vi "Vision Processing.vi"(4 "error in (no error)":errorcluster) -> ()   [LabVIEW 2011]
doc: "This VI runs in parallel to other tasks. It gets images from the camera, processes them for color or shape and use that information to affect robot behavior."
uses:
  <vilib>/Rock Robotics/WPI/Camera/WPI_CameraImageSize.ctl
  <vilib>/Rock Robotics/WPI/Camera/WPI_CameraFrameRate.ctl
  <vilib>/Rock Robotics/WPI/Camera/WPI_CameraExposure Priority Values.ctl
  <vilib>/Rock Robotics/WPI/Camera/WPI_CameraExposure Values.ctl
  <vilib>/Rock Robotics/WPI/Camera/WPI_CameraWhite Balance Values.ctl
  Robot Global Data.vi
  <vilib>/Rock Robotics/WPI/RobotDrive/WPI_RobotDriveArcadeDrive_Standard(NoSaturation).vi
  <vilib>/vision/NI_Vision_Development_Module.lvlib
panel:
  out "max index(es)":i32[](array[numeric])
  out "Loop Speed":u32(knob) scale=100.0..1000.0
  out "Distance":dbl(graph)
  out "Y Error":dbl(graph)
  out "Distance":dbl
  in  "Servo Tilt Gain":dbl=100.0
  out "error out":errorcluster
  out "ServoPosition":dbl
  out "Image Size":T1
  out "X Error":dbl(graph)
  out "X Error":dbl
  in  "Turning Gain":dbl=0.01
  in  "Tracking?":bool
  out "Particle Measurements (Pixels)":dbl[][](array[numeric]) format="%.2f"
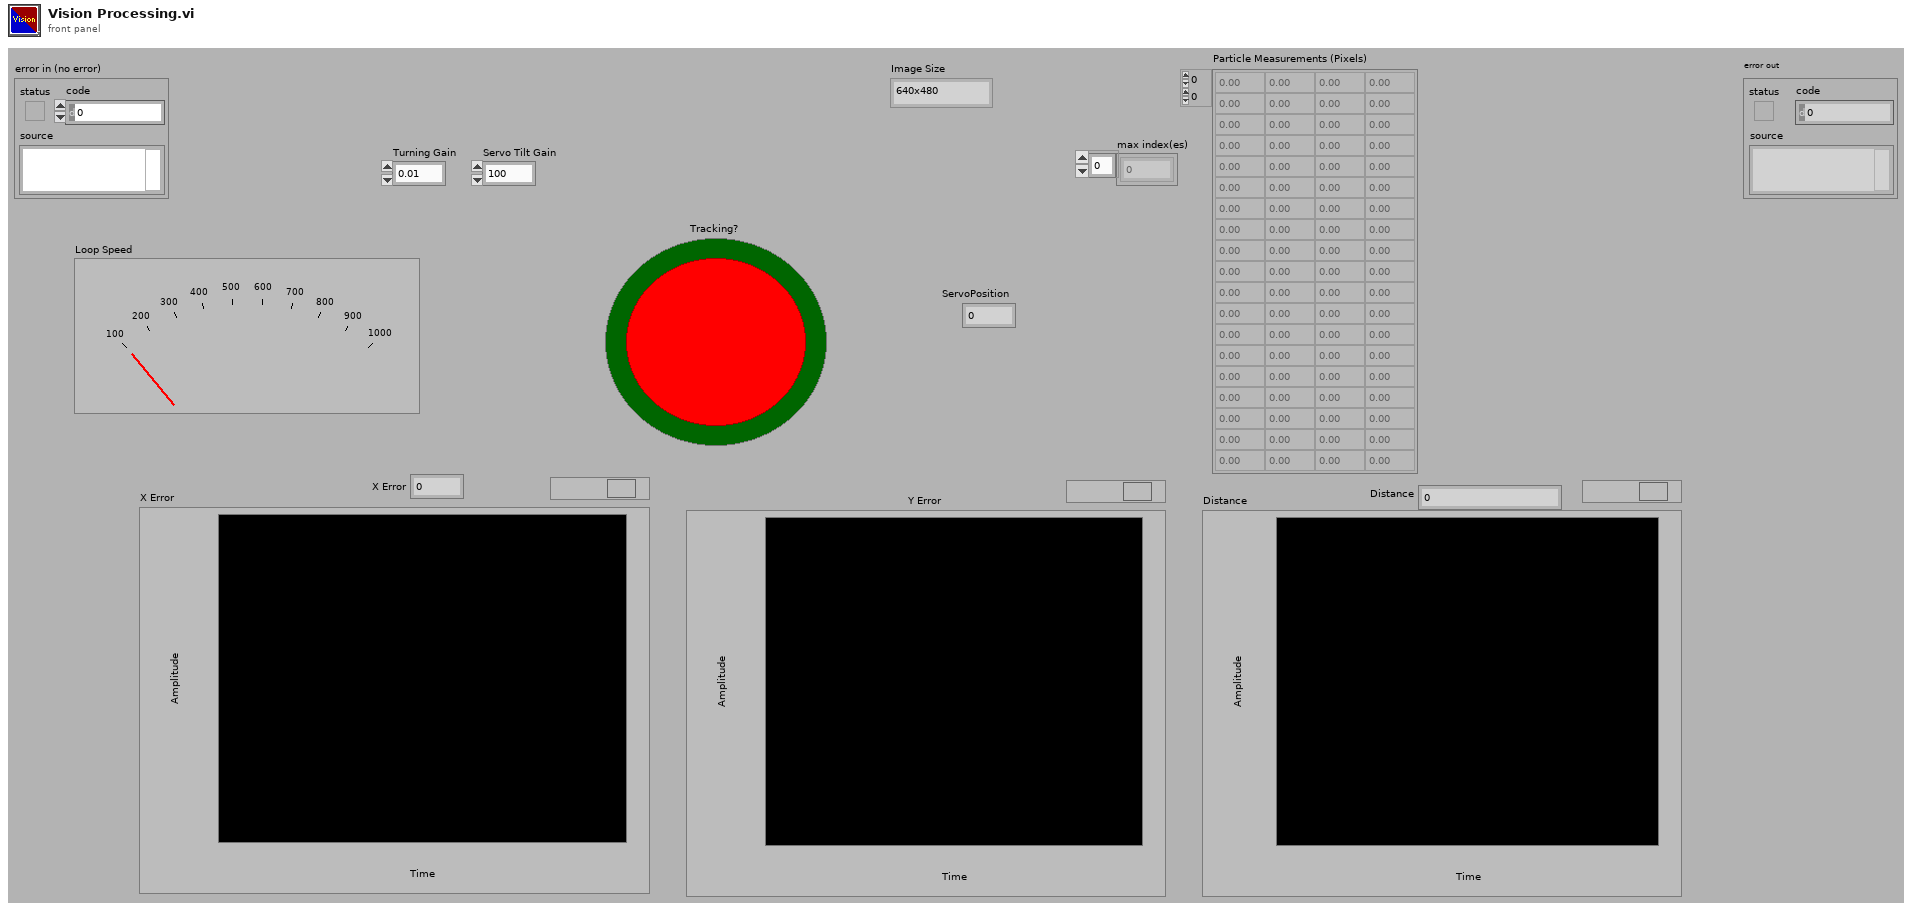
[diagram p1: front panel]
types:
  T1 = typedef "WPI_CameraImageSize.ctl" = enum16{"640x480", "320x240", "160x120"}
  T2 = typedef "Image Type" = u32
  T3 = typedef "WPI_CameraDevRef.ctl" = cluster{"Camera Address":string, "CameraStatus":errorcluster, "Acquire Image Notifier":refnum<notifier>}
  T4 = typedef "WPI_ServoDeviceRef.ctl" = cluster{"DeviceStatus":errorcluster, "Digital Module":T5, "PWM Channel":T6, "DeadBand":T7}
  T5 = typedef "FPGA_TypedefDigitalModule.ctl" = enum16{"Digital Module 1", "Digital Module 2"}
  T6 = typedef "FPGA_DIOPWMChannel.ctl" = enum8{"PWM 1", "PWM 2", "PWM 3", "PWM 4", "PWM 5", "PWM 6", "PWM 7", "PWM 8", "PWM 9", "PWM 10", "Invalid"}
  T7 = typedef "WPI_PWMDeadband.ctl" = cluster{"Name":string, "maxPositivePwm":i32, "minPositivePwm":i32, "centerPwm":i32, "maxNegativePwm":i32, "minNegativePwm":i32, "angularRange":u16}
  T8 = typedef "IMAQ Image.ctl" = refnum<image>
  T9 = enum32{"AutoM", "Close", "Dilate", "Erode", "Gradient", "Gradient out", "Gradient in", "Hit miss", "Open", "PClose", "POpen", "Thick", "Thin"}
  T10 = typedef "WPI_CameraFrameRate.ctl" = u32
  T11 = typedef "WPI_CameraExposure Priority Values.ctl" = enum16{"None", "Prioritize frame rate", "Prioritize image quality"}
  T12 = typedef "WPI_CameraExposure Values.ctl" = enum16{"Auto", "Flicker-free 50 Hz", "Flicker-free 60 Hz", "Hold current"}
  T13 = typedef "WPI_CameraWhite Balance Values.ctl" = enum16{"Auto", "Fixed indoor", "Fixed outdoor 1", "Fixed outdoor 2", "Fixed fluorescent 1", "Fixed fluorescent 2", "Hold current"}
  T14 = typedef "WPI_RobotDriveDevRef.ctl" = cluster{"DevStatus":errorcluster, "Motors[]":T15[], "Square Inputs":bool, "Max Output":dbl, "Isochronous":bool}
  T15 = typedef "WPI_MotorControlDeviceRef.ctl" = cluster{"DeviceStatus":errorcluster, "Type":enum16{"PWM", "CAN"}, "PWM":cluster{"Digital Module":T5, "PWM Channel":T6, "DeadBand":T7}, "CAN":cluster{"Device Number":u8, "Control Mode":T16, "Semaphore":T17, "Max Vout":dbl}, "Invert":bool, "TransformRef":T18, "InvTransformRef":T18}
  T16 = typedef "WPI_CANJaguar_ControlMode.ctl" = enum8{"Percent VBus", "Current", "Speed", "Position", "Voltage"}
  T17 = typedef "Semaphore RefNum" = refnum<k1>
  T18 = typedef "WPI_PWMTransform_ConPane.ctl" = refnum<vi>
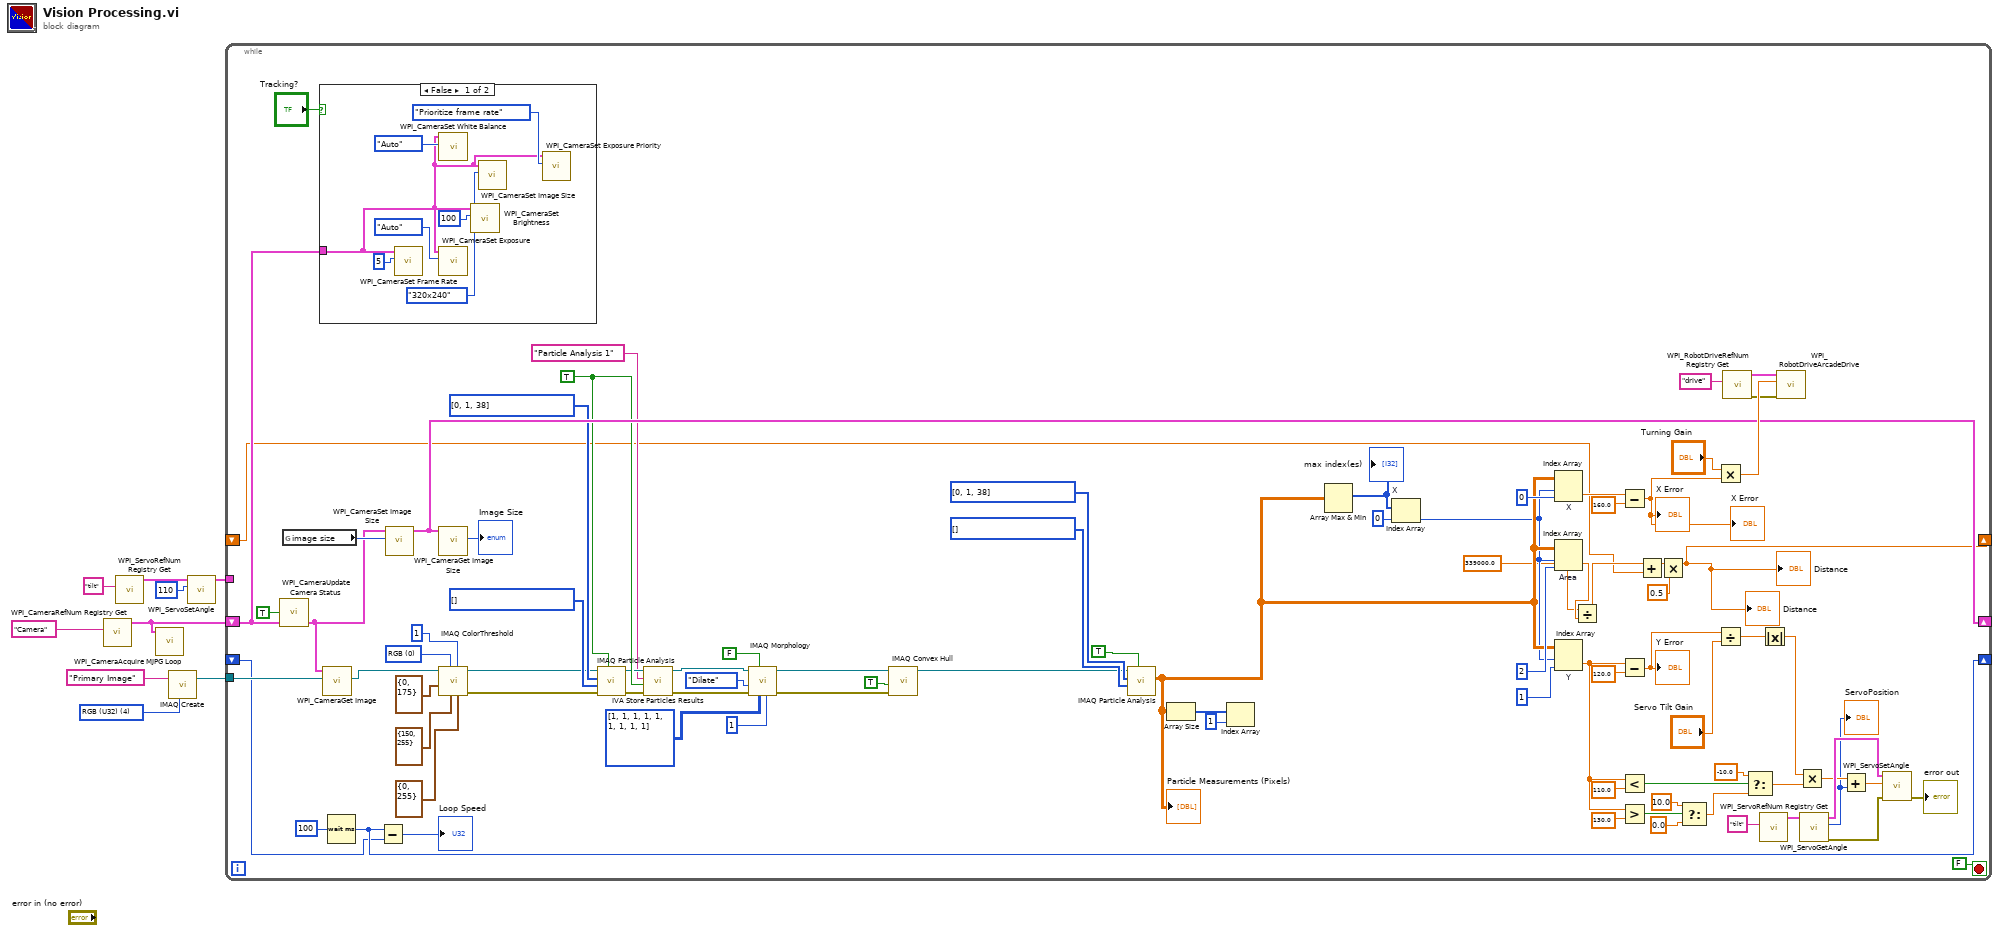
[diagram p0: block diagram]
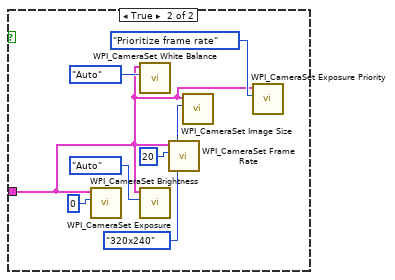
[diagram p2: hidden frame]
diagram:
  w9 = T2 4 items=["Grayscale (U8)", "Grayscale (I16)", "Grayscale (SGL)", "Complex (CSG)", "RGB (U32)", "HSL (U32)", "RGB (U64)"] ("Image Type")
  n1 = call <vilib>:"WPI_CameraRefNum Registry Get.vi"("refnum name"="Camera") -> ("CameraDevRef"=w5:T3)  [unwired: 1 in, 9 out]
  n2 = call <vilib>:"WPI_ServoRefNum Registry Get.vi"("refnum name"="tilt") -> ("ServoDeviceRef"=w2:T4)  [unwired: 9 in, 1 out]
  n3 = call <vilib>:"WPI_CameraAcquire MJPG Loop.vi"("CameraDevRef"=w5) -> ()  [unwired: 11 in]
  n4 = call "IMAQ Create"("Image Name"="Primary Image", "Image Type"=w9) -> ("New Image"=w7:T8)  [unwired: 2 in, 2 out]
  n5 = call <vilib>:"WPI_ServoSetAngle.vi"("Angle"=110, "ServoDeviceRef"=w2) -> ("ServoDeviceRef"=w1:T4)  [unwired: 8 in, 1 out]
  n6 = while {
    shift-right: [w74] -> _
    shift-left: w5 -> [w93]
    tunnel: w7 -> [w73]
    tunnel: w1 -> [_]
    shift-right: [w50] -> _
    shift-left: _ -> [w49]
    shift-right: [w12] -> _
    shift-left: _ -> [w10]
    stop <- FALSE stop-if-true
    w24 = i32[] [] items=["Center of Mass X", "Center of Mass Y", "First Pixel X", "First Pixel Y", "Bounding Rect Left", "Bounding Rect Top", "Bounding Rect Right", "Bounding Rect Bottom", "Max Feret Diameter Start X", "Max Feret Diameter Start Y", "Max Feret Diameter End X", "Max Feret Diameter End Y", "Max Horiz. Segment Length Left", "Max Horiz. Segment Length Right", "Max Horiz. Segment Length Row", "-", "Bounding Rect Width", "Bounding Rect Height", "Bounding Rect Diagonal", "Perimeter", "Convex Hull Perimeter", "Holes' Perimeter", "Max Feret Diameter", "Equivalent Ellipse Major Axis", "Equivalent Ellipse Minor Axis", "Equivalent Ellipse Minor Axis (Feret)", "Equivalent Rect Long Side", "Equivalent Rect Short Side", "Equivalent Rect Diagonal", "Equivalent Rect Short Side (Feret)", "Average Horiz. Segment Length", "Average Vert. Segment Length", "Hydraulic Radius", "Waddel Disk Diameter", "-", "Area", "Holes' Area", "Particle & Holes' Area", "Convex Hull Area", "Image Area", "-", "Number of Holes", "Number of Horiz. Segments", "Number of Vert. Segments", "-", "Orientation", "Max Feret Diameter Orientation", "-", "% Area/Image Area", "% Area/(Particle & Holes' Area)", "Ratio of Equivalent Ellipse Axes", "Ratio of Equivalent Rect Sides", "-", "Elongation Factor", "Compactness Factor", "Heywood Circularity Factor", "Type Factor", "-", "Sum X", "Sum Y", "Sum XX", "Sum XY", "Sum YY", "Sum XXX", "Sum XXY", "Sum XYY", "Sum YYY", "-", "Moment of Inertia XX", "Moment of Inertia XY", "Moment of Inertia YY", "Moment of Inertia XXX", "Moment of Inertia XXY", "Moment of Inertia XYY", "Moment of Inertia YYY", "Norm. Moment of Inertia XX", "Norm. Moment of Inertia XY", "Norm. Moment of Inertia YY", "Norm. Moment of Inertia XXX", "Norm. Moment of Inertia XXY", "Norm. Moment of Inertia XYY", "Norm. Moment of Inertia YYY", "Hu Moment 1", "Hu Moment 2", "Hu Moment 3", "Hu Moment 4", "Hu Moment 5", "Hu Moment 6", "Hu Moment 7"] ("Real-World Measurements")
    w25 = i32[] [0, 1, 38] items=["Center of Mass X", "Center of Mass Y", "First Pixel X", "First Pixel Y", "Bounding Rect Left", "Bounding Rect Top", "Bounding Rect Right", "Bounding Rect Bottom", "Max Feret Diameter Start X", "Max Feret Diameter Start Y", "Max Feret Diameter End X", "Max Feret Diameter End Y", "Max Horiz. Segment Length Left", "Max Horiz. Segment Length Right", "Max Horiz. Segment Length Row", "-", "Bounding Rect Width", "Bounding Rect Height", "Bounding Rect Diagonal", "Perimeter", "Convex Hull Perimeter", "Holes' Perimeter", "Max Feret Diameter", "Equivalent Ellipse Major Axis", "Equivalent Ellipse Minor Axis", "Equivalent Ellipse Minor Axis (Feret)", "Equivalent Rect Long Side", "Equivalent Rect Short Side", "Equivalent Rect Diagonal", "Equivalent Rect Short Side (Feret)", "Average Horiz. Segment Length", "Average Vert. Segment Length", "Hydraulic Radius", "Waddel Disk Diameter", "-", "Area", "Holes' Area", "Particle & Holes' Area", "Convex Hull Area", "Image Area", "-", "Number of Holes", "Number of Horiz. Segments", "Number of Vert. Segments", "-", "Orientation", "Max Feret Diameter Orientation", "-", "% Area/Image Area", "% Area/(Particle & Holes' Area)", "Ratio of Equivalent Ellipse Axes", "Ratio of Equivalent Rect Sides", "-", "Elongation Factor", "Compactness Factor", "Heywood Circularity Factor", "Type Factor", "-", "Sum X", "Sum Y", "Sum XX", "Sum XY", "Sum YY", "Sum XXX", "Sum XXY", "Sum XYY", "Sum YYY", "-", "Moment of Inertia XX", "Moment of Inertia XY", "Moment of Inertia YY", "Moment of Inertia XXX", "Moment of Inertia XXY", "Moment of Inertia XYY", "Moment of Inertia YYY", "Norm. Moment of Inertia XX", "Norm. Moment of Inertia XY", "Norm. Moment of Inertia YY", "Norm. Moment of Inertia XXX", "Norm. Moment of Inertia XXY", "Norm. Moment of Inertia XYY", "Norm. Moment of Inertia YYY", "Hu Moment 1", "Hu Moment 2", "Hu Moment 3", "Hu Moment 4", "Hu Moment 5", "Hu Moment 6", "Hu Moment 7"] ("Pixel Measurements")
    w40 = i32[] [] items=["Center of Mass X", "Center of Mass Y", "First Pixel X", "First Pixel Y", "Bounding Rect Left", "Bounding Rect Top", "Bounding Rect Right", "Bounding Rect Bottom", "Max Feret Diameter Start X", "Max Feret Diameter Start Y", "Max Feret Diameter End X", "Max Feret Diameter End Y", "Max Horiz. Segment Length Left", "Max Horiz. Segment Length Right", "Max Horiz. Segment Length Row", "-", "Bounding Rect Width", "Bounding Rect Height", "Bounding Rect Diagonal", "Perimeter", "Convex Hull Perimeter", "Holes' Perimeter", "Max Feret Diameter", "Equivalent Ellipse Major Axis", "Equivalent Ellipse Minor Axis", "Equivalent Ellipse Minor Axis (Feret)", "Equivalent Rect Long Side", "Equivalent Rect Short Side", "Equivalent Rect Diagonal", "Equivalent Rect Short Side (Feret)", "Average Horiz. Segment Length", "Average Vert. Segment Length", "Hydraulic Radius", "Waddel Disk Diameter", "-", "Area", "Holes' Area", "Particle & Holes' Area", "Convex Hull Area", "Image Area", "-", "Number of Holes", "Number of Horiz. Segments", "Number of Vert. Segments", "-", "Orientation", "Max Feret Diameter Orientation", "-", "% Area/Image Area", "% Area/(Particle & Holes' Area)", "Ratio of Equivalent Ellipse Axes", "Ratio of Equivalent Rect Sides", "-", "Elongation Factor", "Compactness Factor", "Heywood Circularity Factor", "Type Factor", "-", "Sum X", "Sum Y", "Sum XX", "Sum XY", "Sum YY", "Sum XXX", "Sum XXY", "Sum XYY", "Sum YYY", "-", "Moment of Inertia XX", "Moment of Inertia XY", "Moment of Inertia YY", "Moment of Inertia XXX", "Moment of Inertia XXY", "Moment of Inertia XYY", "Moment of Inertia YYY", "Norm. Moment of Inertia XX", "Norm. Moment of Inertia XY", "Norm. Moment of Inertia YY", "Norm. Moment of Inertia XXX", "Norm. Moment of Inertia XXY", "Norm. Moment of Inertia XYY", "Norm. Moment of Inertia YYY", "Hu Moment 1", "Hu Moment 2", "Hu Moment 3", "Hu Moment 4", "Hu Moment 5", "Hu Moment 6", "Hu Moment 7"] ("Real-World Measurements")
    w41 = i32[] [0, 1, 38] items=["Center of Mass X", "Center of Mass Y", "First Pixel X", "First Pixel Y", "Bounding Rect Left", "Bounding Rect Top", "Bounding Rect Right", "Bounding Rect Bottom", "Max Feret Diameter Start X", "Max Feret Diameter Start Y", "Max Feret Diameter End X", "Max Feret Diameter End Y", "Max Horiz. Segment Length Left", "Max Horiz. Segment Length Right", "Max Horiz. Segment Length Row", "-", "Bounding Rect Width", "Bounding Rect Height", "Bounding Rect Diagonal", "Perimeter", "Convex Hull Perimeter", "Holes' Perimeter", "Max Feret Diameter", "Equivalent Ellipse Major Axis", "Equivalent Ellipse Minor Axis", "Equivalent Ellipse Minor Axis (Feret)", "Equivalent Rect Long Side", "Equivalent Rect Short Side", "Equivalent Rect Diagonal", "Equivalent Rect Short Side (Feret)", "Average Horiz. Segment Length", "Average Vert. Segment Length", "Hydraulic Radius", "Waddel Disk Diameter", "-", "Area", "Holes' Area", "Particle & Holes' Area", "Convex Hull Area", "Image Area", "-", "Number of Holes", "Number of Horiz. Segments", "Number of Vert. Segments", "-", "Orientation", "Max Feret Diameter Orientation", "-", "% Area/Image Area", "% Area/(Particle & Holes' Area)", "Ratio of Equivalent Ellipse Axes", "Ratio of Equivalent Rect Sides", "-", "Elongation Factor", "Compactness Factor", "Heywood Circularity Factor", "Type Factor", "-", "Sum X", "Sum Y", "Sum XX", "Sum XY", "Sum YY", "Sum XXX", "Sum XXY", "Sum XYY", "Sum YYY", "-", "Moment of Inertia XX", "Moment of Inertia XY", "Moment of Inertia YY", "Moment of Inertia XXX", "Moment of Inertia XXY", "Moment of Inertia XYY", "Moment of Inertia YYY", "Norm. Moment of Inertia XX", "Norm. Moment of Inertia XY", "Norm. Moment of Inertia YY", "Norm. Moment of Inertia XXX", "Norm. Moment of Inertia XXY", "Norm. Moment of Inertia XYY", "Norm. Moment of Inertia YYY", "Hu Moment 1", "Hu Moment 2", "Hu Moment 3", "Hu Moment 4", "Hu Moment 5", "Hu Moment 6", "Hu Moment 7"] ("Pixel Measurements")
    w38 = TRUE ("Connectivity 4/8 (8)")
    w46 = u16 0 items=["RGB", "HSL", "HSV", "HSI"] ("Color Mode")
    n7 = call <vilib>:"WPI_CameraUpdate Camera Status.vi"("CameraDevRef In"=w93, "Enable Vision"=TRUE) -> ("CameraDevRef Out"=w72:T3)  [unwired: 3 in]
    n8 = global read "Robot Global Data.vi" "image size"() -> (w92:T1)
    n9 = case shown="False" "Tracking?" {
      tunnel: w93 -> [w97 w105]
      frame False {
        n10 = call <vilib>:"WPI_CameraSet Frame Rate.vi"("Frame Rate (fps)"=T10 5, "CameraDevRef"=w97) -> ()  [unwired: 8 in, 2 out]
        n11 = call <vilib>:"WPI_CameraSet White Balance.vi"("White Balance"=WPI_CameraWhite_Balance_Values."Auto", "CameraDevRef"=w97) -> ()  [unwired: 8 in, 2 out]
        n12 = call <vilib>:"WPI_CameraSet Exposure.vi"("Exposure"=WPI_CameraExposure_Values."Auto", "CameraDevRef"=w97) -> ()  [unwired: 8 in, 2 out]
        n13 = call <vilib>:"WPI_CameraSet Brightness.vi"("Brightness"=100, "CameraDevRef"=w97) -> ()  [unwired: 8 in, 2 out]
        n14 = call <vilib>:"WPI_CameraSet Image Size.vi"("Image Size"=WPI_CameraImageSize."320x240", "CameraDevRef"=w97) -> ()  [unwired: 8 in, 2 out]
        n15 = call <vilib>:"WPI_CameraSet Exposure Priority.vi"("Exposure Priority"=WPI_CameraExposure_Priority_Values."Prioritize frame rate", "CameraDevRef"=w97) -> ()  [unwired: 8 in, 2 out]
      }
      frame True {
        n16 = call <vilib>:"WPI_CameraSet Brightness.vi"("Brightness"=0, "CameraDevRef"=w105) -> ()  [unwired: 8 in, 2 out]
        n17 = call <vilib>:"WPI_CameraSet White Balance.vi"("White Balance"=WPI_CameraWhite_Balance_Values."Auto", "CameraDevRef"=w105) -> ()  [unwired: 8 in, 2 out]
        n18 = call <vilib>:"WPI_CameraSet Exposure.vi"("Exposure"=WPI_CameraExposure_Values."Auto", "CameraDevRef"=w105) -> ()  [unwired: 8 in, 2 out]
        n19 = call <vilib>:"WPI_CameraSet Frame Rate.vi"("Frame Rate (fps)"=T10 20, "CameraDevRef"=w105) -> ()  [unwired: 8 in, 2 out]
        n20 = call <vilib>:"WPI_CameraSet Image Size.vi"("Image Size"=WPI_CameraImageSize."320x240", "CameraDevRef"=w105) -> ()  [unwired: 8 in, 2 out]
        n21 = call <vilib>:"WPI_CameraSet Exposure Priority.vi"("Exposure Priority"=WPI_CameraExposure_Priority_Values."Prioritize frame rate", "CameraDevRef"=w105) -> ()  [unwired: 8 in, 2 out]
      }
    }
    n22 = call <vilib>:"WPI_CameraGet Image.vi"("Image"=w73, "CameraDevRef"=w72) -> ("Image Out"=w22:T8)  [unwired: 7 in, 2 out]
    n23 = Wait (ms)(milliseconds to wait=u32 100) -> (millisecond timer value=w50:u32)
    n24 = Subtract(x=w50, y=w49) -> (x-y=→"Loop Speed":u32)
    n25 = call <vilib>:"WPI_CameraSet Image Size.vi"("Image Size"=w92, "CameraDevRef"=w72) -> ("CameraDevRef Out"=w74:T3)  [unwired: 1 in, 8 out]
    n26 = call <vilib>:"WPI_CameraGet Image Size.vi"("CameraDevRef"=w74) -> ("Image Size"=→"Image Size":T1)  [unwired: 8 in, 2 out]
    n27 = call "IMAQ ColorThreshold"("Blue or Luma or Val or Inten Range"=cluster{"Lower value":i32, "Upper value":i32} {"Lower value"=0, "Upper value"=255}, "Replace Value"=1, "Green or Sat Range"=cluster{"Lower value":i32, "Upper value":i32} {"Lower value"=150, "Upper value"=255}, "Color Mode"=w46, "Red or Hue Range"=cluster{"Lower value":i32, "Upper value":i32} {"Lower value"=0, "Upper value"=175}, "Image Src"=w22) -> ("error out"=w42:errorcluster, "Image Dst Out"=w39:T8)  [unwired: 2 in, 2 out]
    n28 = call "IMAQ Particle Analysis"("Connectivity 4/8 (8)"=w38, "error in (no error)"=w42, "Real-World Measurements"=w40, "Pixel Measurements"=w41, "Image"=w39) -> ("error out"=w35:errorcluster, "Image Out (duplicate)"=w37:T8)  [unwired: 5 out]
    n29 = call <vilib>:"IVA Store Particles Results.vi"("error in (no error)"=w35, "Connectivity 4/8 (8)"=w38, "Step Name"="Particle Analysis 1", "Image in"=w37) -> ("error out"=w34:errorcluster, "Image dup"=w29:T8)  [unwired: 6 out]
    n30 = call "IMAQ Morphology"("Number of iterations (1)"=1, "Structuring Element"=i32[][] [[1, 1, 1], [1, 1, 1], [1, 1, 1]], "Square/Hexa (Square)"=FALSE, "error in (no error)"=w34, "Operation"=T9."Dilate", "Image Src"=w29) -> ("error out"=w28:errorcluster, "Image Dst Out"=w27:T8)  [unwired: 1 in, 3 out]
    n31 = call "IMAQ Convex Hull"("error in (no error)"=w28, "Connectivity 4/8 (8)"=TRUE, "Image Src"=w27) -> ("Image Dst Out"=w21:T8)  [unwired: 1 in, 7 out]
    n32 = call "IMAQ Particle Analysis"("Connectivity 4/8 (8)"=TRUE, "Real-World Measurements"=w24, "Pixel Measurements"=w25, "Image"=w21) -> ("Particle Measurements (Pixels)"=w20:dbl[][])  [unwired: 1 in, 6 out]
    "Particle Measurements (Pixels)" <- w20
    n33 = Array Size(array=w20) -> (size(s)=w91:i32[])
    n34 = Index Array(array=w91, index=1) -> ()  [unwired: 1 out]
    n35 = Array Max & Min(array=w20) -> (max index (indices)=w19:i32[])  [unwired: 3 out]
    "max index(es)" <- w19
    n36 = Index Array "X"(array=w19, index=0) -> (element=w17:i32)
    n37 = Index Array "X"(array=w20, index (row)=w17, index (col)=0 ("disabled index (col)")) -> (element=w87:dbl)
    n38 = Index Array "Area"(array=w20, index (row)=w17, index (col)=2 ("disabled index (col)")) -> (element=w15:dbl)
    n39 = Index Array "Y"(array=w20, index (row)=w17, index (col)=1 ("disabled index (col)")) -> (element=w57:dbl)
    n40 = Divide(x=339000.0 ("Factor"), y=w15) -> (x/y=w16:dbl)
    n41 = Subtract(x=w87, y=160.0) -> (x-y=w78:dbl)
    "X Error" <- w78
    "X Error" <- w78
    n42 = Subtract(x=w57, y=120.0) -> (x-y=w51:dbl)
    "Y Error" <- w51
    n43 = Less?(x=w57, y=110.0) -> (x < y?=w67:bool)
    n44 = Greater?(x=w57, y=130.0) -> (0:w66:bool)
    n45 = Add(x=w16, y=w10) -> (x+y=w13:dbl)
    n46 = Multiply(x=w13, y=0.5) -> (x*y=w12:dbl)
    "Distance" <- w12
    "Distance" <- w12
    n47 = Select(t=10.0, s=w66, f=0.0) -> (s? t:f=w65:dbl)
    n48 = Multiply(x="Turning Gain", y=w78) -> (x*y=w83:dbl)
    n49 = Divide(x=w51, y="Servo Tilt Gain") -> (x/y=w55:dbl)
    n50 = call <vilib>:"WPI_RobotDriveRefNum Registry Get.vi"("refnum name"="drive") -> ("error out"=w75:errorcluster, "RobotDriveDevRef"=w84:T14)  [unwired: 9 in]
    n51 = Select(t=-10.0, s=w67, f=w65) -> (s? t:f=w62:dbl)
    n52 = call <vilib>:"WPI_ServoRefNum Registry Get.vi"("refnum name"="tilt") -> ("ServoDeviceRef"=w81:T4)  [unwired: 9 in, 1 out]
    n53 = Absolute Value(x=w55) -> (abs(x)=w54:dbl)
    n54 = call-poly <vilib>:"WPI_RobotDriveArcadeDrive.vi"("error in (no error)"=w75, "X axis value"=w83, "RobotDriveDevRef"=w84) -> ()  [unwired: 7 in, 2 out]
    n55 = Multiply(x=w54, y=w62) -> (x*y=w61:dbl)
    n56 = call <vilib>:"WPI_ServoGetAngle.vi"("ServoDeviceRef"=w81) -> ("ServoDeviceRef"=w79:T4, "Angle"=w52:u16, "error out"=w71:errorcluster)  [unwired: 7 in]
    "ServoPosition" <- w52
    n57 = Add(x=w61, y=w52) -> (x+y=w59:dbl)
    n58 = call <vilib>:"WPI_ServoSetAngle.vi"("error in (no error)"=w71, "Angle"=w59, "ServoDeviceRef"=w79) -> ("error out"=→"error out":errorcluster)  [unwired: 7 in, 1 out]
  }
